vi "Convert.vi"(0 "Данные с прибора":string) -> (1 "Емкость":dbl, 2 "Потери":dbl)   [LabVIEW 2016]
panel:
  out "munpF":string
  out "MAIN:SECO":string
  out "SECO Value":string
  out "SECO VALUE":string
  out "MAIN:PRIM":string
  out "PRIM Value":string
  out "PRIM VALUE":string
  out "Numeric PRIM":dbl
  out "Результаты измерения":string
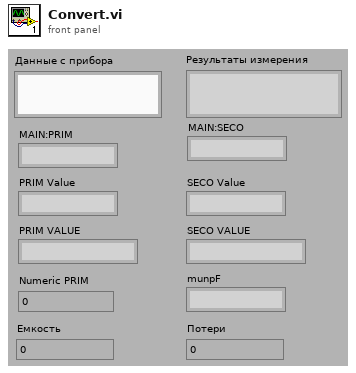
[diagram p1: front panel]
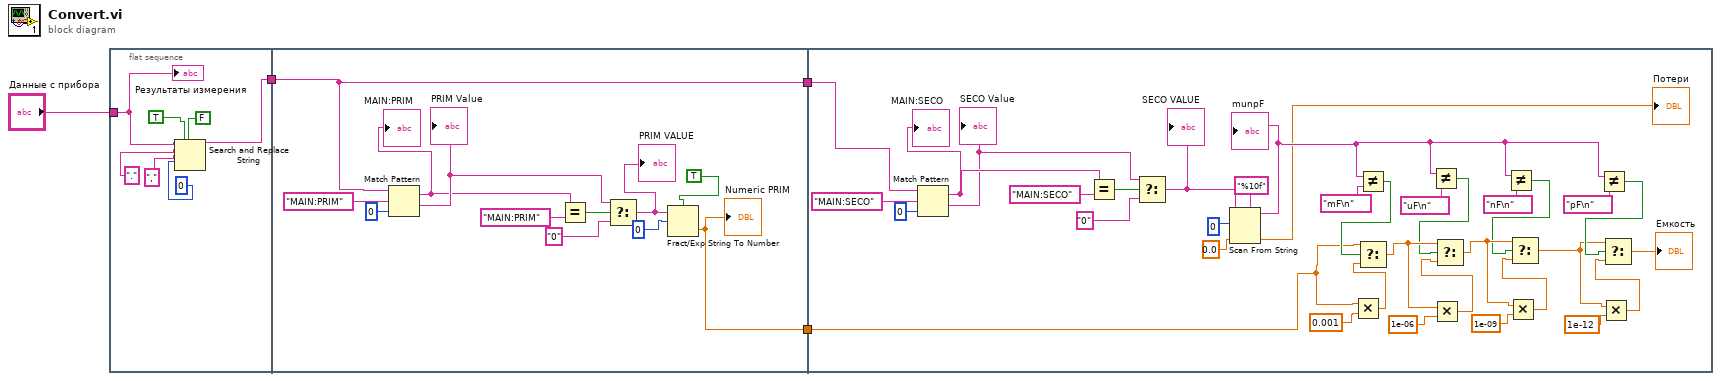
[diagram p0: block diagram]
diagram:
  n1 = flat-sequence {
    tunnel: [w7] -> w4
    tunnel: "Данные с прибора" -> [w5]
    tunnel: [w13] -> w3
    tunnel: [w12] -> w2
    tunnel: w4 -> [w12]
    tunnel: w3 -> [w27]
    tunnel: w2 -> [w47]
    frame #0 {
      n2 = Search and Replace String(replace all?=TRUE, case sensitive?=FALSE, input string=w5, search string=".", replace string=",", offset=0) -> (result string=w7:string)  [unwired: 2 in, 3 out]
      "Результаты измерения" <- w5
    }
    frame #1 {
      n3 = Match Pattern(string=w12, regular expression="MAIN:PRIM", offset (0)=0) -> (match substring=w18:string, after substring=w19:string)  [unwired: 2 out]
      "MAIN:PRIM" <- w18
      "PRIM Value" <- w19
      n4 = Equal?(x=w18, y="MAIN:PRIM") -> (x = y?=w20:bool)
      n5 = Select(t=w19, s=w20, f="0") -> (s? t:f=w16:string)
      "PRIM VALUE" <- w16
      n6 = Fract/Exp String To Number(use system decimal point (T)=TRUE, string=w16, offset=0) -> (number=w13:dbl)  [unwired: 1 in, 1 out]
      "Numeric PRIM" <- w13
    }
    frame #2 {
      n7 = Match Pattern(string=w47, regular expression="MAIN:SECO", offset (0)=0) -> (match substring=w51:string, after substring=w49:string)  [unwired: 2 out]
      "MAIN:SECO" <- w51
      "SECO Value" <- w49
      n8 = Equal?(x=w51, y="MAIN:SECO") -> (x = y?=w52:bool)
      n9 = Select(t=w49, s=w52, f="0") -> (s? t:f=w50:string)
      "SECO VALUE" <- w50
      n10 = Scan From String "Scan From String"(format string="%10f", input string=w50, initial scan location=0, default 1=0.0) -> (remaining string=w26:string, output 1=→"Потери":dbl)  [unwired: 1 in, 2 out]
      "munpF" <- w26
      n11 = Multiply(x=w27, y=0.001) -> (x*y=w46:dbl)
      n12 = Not Equal?(x=w26, y="mF\n") -> (x != y?=w38:bool)
      n13 = Select(t=w27, s=w38, f=w46) -> (s? t:f=w45:dbl)
      n14 = Not Equal?(x=w26, y="uF\n") -> (x != y?=w33:bool)
      n15 = Multiply(x=w45, y=1e-06) -> (x*y=w43:dbl)
      n16 = Select(t=w45, s=w33, f=w43) -> (s? t:f=w44:dbl)
      n17 = Not Equal?(x=w26, y="nF\n") -> (x != y?=w34:bool)
      n18 = Multiply(x=w44, y=1e-09) -> (x*y=w42:dbl)
      n19 = Select(t=w44, s=w34, f=w42) -> (s? t:f=w28:dbl)
      n20 = Not Equal?(x=w26, y="pF\n") -> (x != y?=w29:bool)
      n21 = Multiply(x=w28, y=1e-12) -> (x*y=w32:dbl)
      n22 = Select(t=w28, s=w29, f=w32) -> (s? t:f=→"Емкость":dbl)
    }
  }
